vi "Write Target.vi"(8 "error in (no error)":errorcluster, 10 "State Machine.lvlib:State.lvlib:State.lvclass":refnum<class "State.lvclass">, 11 "Transition in":refnum<class "Transition.lvclass">) -> (0 "error out":errorcluster, 3 "Transition out":refnum<class "Transition.lvclass">)   [LabVIEW 2024, in "Transition.lvlib" / "Transition.lvclass"]
uses:
  Transition.lvclass
  State/State/State.lvclass
  Transition.lvclass/Transition.ctl
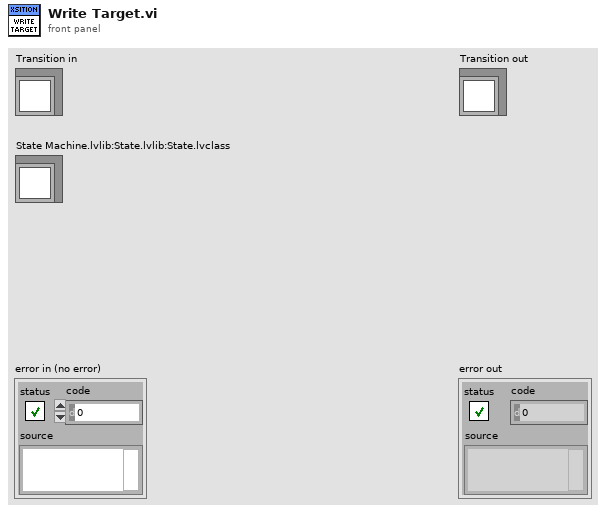
[diagram p1: front panel]
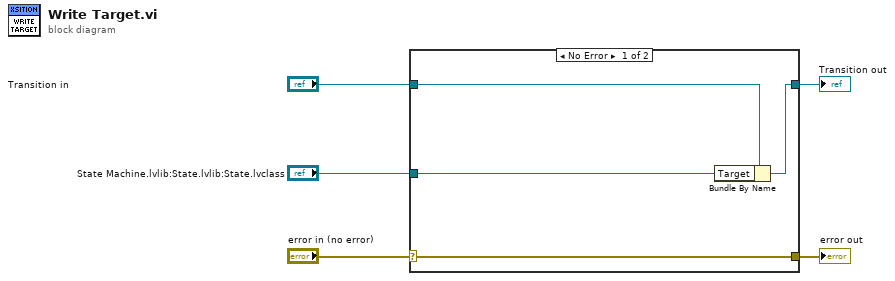
[diagram p0: block diagram]
diagram:
  n1 = case shown="No Error" "error in (no error)" {
    selector: "error in (no error)" -> [w9 w10]
    tunnel: [w9 w10] -> w4
    tunnel: [w7 w11] -> w2
    tunnel: "Transition in" -> [w8 w11]
    tunnel: "State Machine.lvlib:State.lvlib:State.lvclass" -> [w6 _]
    frame No Error {
      n2 = Bundle By Name(cluster=w8, "Target"=w6) -> (w7:refnum<class "Transition.lvclass">)
    }
    frame Error {
    }
  }
  "error out" <- w4
  "Transition out" <- w2
